vi "Set Waveform Display Intensity.vi"(8 "error in (no error)":errorcluster, 10 "Intensity (1-100)":i8=1 min=1 max=100 step=1, 11 "DPO4104 in":refnum<class "DPO4104.lvclass">) -> (0 "error out":errorcluster, 3 "DPO4104 out":refnum<class "DPO4104.lvclass">)   [LabVIEW 2018, in "DPO4104.lvlib" / "DPO4104.lvclass"]
doc: "This Override is used to change the display intensity level for the oscilloscope waveforms."
uses:
  DPO4104.lvclass
  <instrlib>/Tektronix DPO MSO 2000 4000 Series/Tektronix DPO MSO 2000 4000 Series.lvlib
  PPLs/Oscilloscope/Parent/Oscilloscope.lvlibp/Oscilloscope.lvclass
  C:/Projects/LabVIEW/PPLs/Oscilloscope/Parent/Oscilloscope.lvlibp/Oscilloscope.lvclass
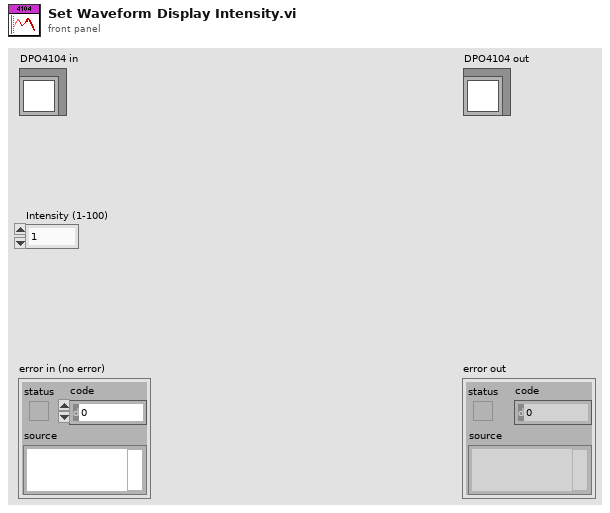
[diagram p1: front panel]
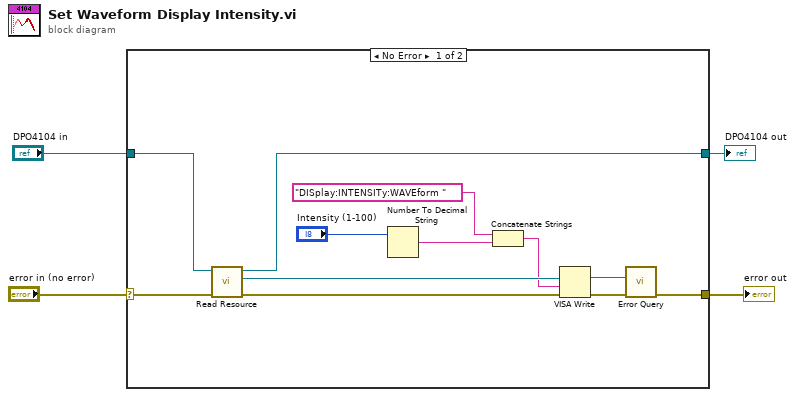
[diagram p0: block diagram]
diagram:
  n1 = case shown="No Error" "error in (no error)" {
    selector: "error in (no error)" -> [w15 w17]
    tunnel: [w11 w17] -> w3
    tunnel: [w9 w18] -> w2
    tunnel: "DPO4104 in" -> [w16 w18]
    frame No Error {
      n2 = call "Read Resource.vi"("error in (no error)"=w15, "Oscilloscope in"=w16) -> ("error out"=w12:errorcluster, "Resource"=w8:refnum<visa-resource-name>, "Oscilloscope out"=w9:refnum<class "DPO4104.lvclass">)  [unwired: 7 in]
      n3 = Number To Decimal String(number="Intensity (1-100)") -> (decimal integer string=w7:string)  [unwired: 1 in]
      n4 = Concatenate Strings("DISplay:INTENSITy:WAVEform ", w7) -> (w5:string)
      n5 = VISA Write(VISA resource name=w8, write buffer=w5, error in (no error)=w12) -> (VISA resource name out=w13:refnum<visa-resource-name>, error out=w14:errorcluster)  [unwired: 1 out]
      n6 = call <instrlib>:"Error Query.vi"("error in (no error)"=w14, "VISA resource name"=w13) -> ("error out"=w11:errorcluster)  [unwired: 6 in, 3 out]
    }
    frame Error {
    }
  }
  "error out" <- w3
  "DPO4104 out" <- w2
